vi "error_raise.vi"(7 "message":string, 8 "error in (no error)":errorcluster, 11 "toml":string) -> (0 "error out":errorcluster)   [LabVIEW 2017, in "toml.lvlib"]
uses:
  toml.lvlib
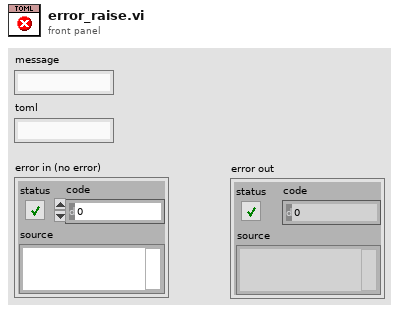
[diagram p1: front panel]
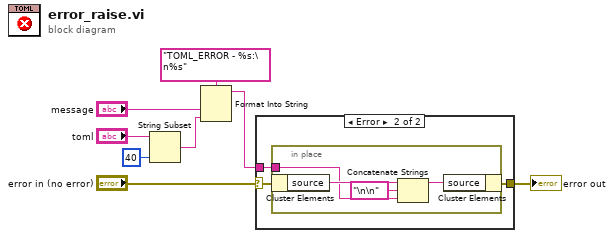
[diagram p0: block diagram]
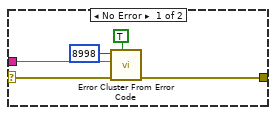
[diagram p2: hidden frame]
diagram:
  n1 = String Subset(string="toml", length (rest)=40 ("length (rest)")) -> (substring=w1:string)  [unwired: 1 in]
  n2 = Format Into String(format string="TOML_ERROR - %s:\n%s" ("error message (\"\")"), "message", w1) -> (resulting string=w6:string)  [unwired: 2 in, 1 out]
  n3 = case shown="Error" "error in (no error)" {
    selector: "error in (no error)" -> [w13 w16]
    tunnel: [w12 w15] -> w7
    tunnel: w6 -> [w9 w14]
    frame No Error {
      n4 = call <vilib>:"Error Cluster From Error Code.vi"("show call chain? (False)"=TRUE, "error in (no error)"=w13, "error message (\"\")"=w9, "error code (0)"=8998) -> ("error out"=w12:errorcluster)  [unwired: 5 in]
    }
    frame Error {
      n5 = in-place {
        in-place-border: w14 -> [w18]
        n6 = in-place-cluster #1(w16) -> ("source"=w20:string)
        n7 = Concatenate Strings(w20, "\n\n" ("string"), w18) -> (w19:string)
        n8 = in-place-cluster #1("source"=w19) -> (w15:errorcluster)
      }
    }
  }
  "error out" <- w7
